vi "Begin.vi"(8 "error in":errorcluster) -> (0 "error out":errorcluster)   [LabVIEW 2015]
doc: "Called before other user functions, this VI is expected to open initial I/O refnums, load in file data, and do all program initialization. Notice that the <B>error out</B> terminal is simply used for data flow. Wiring it to other structures or subVIs ensures that this VI runs first."
uses:
  <vilib>/Rock Robotics/WPI/DriverStation/WPI_DriverStationRobotMode2.ctl
  <vilib>/Rock Robotics/SystemInterfaces/DIO/FPGA_DIOPWMChannel.ctl
  <vilib>/Rock Robotics/WPI/SafetyOutput/WPI_SafetyOutputConfigMenu.ctl
  <vilib>/Rock Robotics/WPI/Joystick/WPI_JoystickDeviceEnum.ctl
  <vilib>/Rock Robotics/WPI/Solenoid/WPI_SolenoidChannel.ctl
  <vilib>/Rock Robotics/SystemInterfaces/DIO/FPGA_DIOChannel.ctl
  <vilib>/Rock Robotics/SystemInterfaces/DIO/FPGA_DIORelayChannel.ctl
  <vilib>/Rock Robotics/SystemInterfaces/spilib/spi_bus.ctl
  Robot Global Data.vi
  <vilib>/Rock Robotics/WPI/RobotDrive/WPI_RobotDriveOpen2MotorWithVictor.vi
  <vilib>/Rock Robotics/WPI/MotorControl/WPI_MotorControlOpen Victor.vi
  <vilib>/Rock Robotics/WPI/MotorControl/WPI_MotorControlOpen SPARK.vi
  <vilib>/Rock Robotics/WPI/Counter/WPI_CounterDigitalInputToDigitalSource.vi
  <vilib>/Rock Robotics/WPI/Counter/WPI_CounterOpen UpDown Mode.vi
  <vilib>/Rock Robotics/WPI/Solenoid/WPI_SolenoidOpenDouble.vi
  <vilib>/Rock Robotics/WPI/Gyro/WPI_GyroXRS450_SPI_Open.vi
  Robot Global.vi
  <vilib>/Rock Robotics/WPI/Accelerometer/InternalAccelerometer/WPI_AccelerometerInternalOpen.vi
  <vilib>/Rock Robotics/SystemInterfaces/AI/FPGA_AIChannel.ctl
  <vilib>/Rock Robotics/Network Tables/NT Write String Array.vi
  <vilib>/Rock Robotics/SystemInterfaces/AI/FPGA_AIGyroChannel.ctl
  <vilib>/Rock Robotics/WPI/Solenoid/WPI_SolenoidOpenSingle.vi
  <vilib>/Rock Robotics/WPI/Ultrasonic/WPI_SonarMB1010AnalogOpen.vi
  <vilib>/Rock Robotics/WPI/Gyro/WPI_GyroAnalogOpen.vi
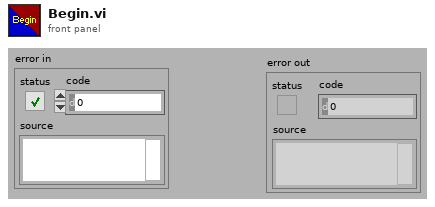
[diagram p1: front panel]
types:
  T1 = typedef "WPI_DriverStationRobotMode2.ctl" = enum16{"Autonomous Disabled", "Autonomous Enabled", "Teleop Disabled", "Teleop Enabled", "Disconnected", "Finish", "Test Disabled", "Test Enabled", "Emergency Stopped"}
  T2 = typedef "FPGA_DIOChannel.ctl" = enum8{"DIO 0", "DIO 1", "DIO 2", "DIO 3", "DIO 4", "DIO 5", "DIO 6", "DIO 7", "DIO 8", "DIO 9", "DIO MXP 0", "DIO MXP 1", "DIO MXP 2", "DIO MXP 3", "DIO MXP 4", "DIO MXP 5", "DIO MXP 6", "DIO MXP 7", "DIO MXP 8", "DIO MXP 9", "DIO MXP 10", "DIO MXP 11", "DIO MXP 12", "DIO MXP 13", "DIO MXP 14", "DIO MXP 15", "Invalid"}
  T3 = typedef "FPGA_DIOPWMChannel.ctl" = enum8{"PWM 0", "PWM 1", "PWM 2", "PWM 3", "PWM 4", "PWM 5", "PWM 6", "PWM 7", "PWM 8", "PWM 9", "PWM MXP 0", "PWM MXP 1", "PWM MXP 2", "PWM MXP 3", "PWM MXP 4", "PWM MXP 5", "PWM MXP 6", "PWM MXP 7", "PWM MXP 8", "PWM MXP 9", "Invalid"}
  T4 = typedef "FPGA_AIChannel.ctl" = enum8{"AI 0", "AI 1", "AI 2", "AI 3", "AI MXP 0", "AI MXP 1", "AI MXP 2", "AI MXP 3", "Invalid"}
  T5 = typedef "WPI_JoystickDeviceEnum.ctl" = enum16{"USB 0", "USB 1", "USB 2", "USB 3", "USB 4", "USB 5"}
  T6 = typedef "WPI_SolenoidChannel.ctl" = enum8{"Solenoid 0", "Solenoid 1", "Solenoid 2", "Solenoid 3", "Solenoid 4", "Solenoid 5", "Solenoid 6", "Solenoid 7", "Invalid"}
  T7 = typedef "FPGA_AIGyroChannel.ctl" = enum8{"AI 0", "AI 1", "Invalid"}
  T8 = typedef "WPI_SafetyOutputConfigMenu.ctl" = enum16{"Enable", "Disable"}
  T9 = typedef "spi_bus.ctl" = enum16{"SPI On-Board, CS0", "SPI On-Board, CS1", "SPI On-Board, CS2", "SPI On-Board, CS3", "SPI MXP", "Invalid"}
  T10 = typedef "FPGA_DIORelayChannel.ctl" = enum8{"Relay 0", "Relay 1", "Relay 2", "Relay 3", "Invalid"}
  T11 = typedef "WPI_SolenoidDevRef.ctl" = cluster{"DevStatus":errorcluster, "Pneumatics Control Module":u8, "Forward Solenoid Channel":T6, "Reverse Solenoid Channel":T6}
  T12 = typedef "WPI_DigitalInputDevRef.ctl" = cluster{"DevStatus":errorcluster, "DIO Channel":T2}
  T13 = typedef "WPI_CompressorDevRef.ctl" = cluster{"DevStatus":errorcluster, "Pneumatics Control Module":u8}
  T14 = typedef "FPGA_CounterEncoderSourceConvertionLVSourceType.ctl" = cluster{"DevStatus":errorcluster, "AnalogTriggerMode?":bool, "DigitalMode":cluster{"DIO Channel":T15}, "AnalogTriggerMode":cluster{"AnalogTriggerIndex":T16, "OutputType":T17}}
  T15 = typedef "FPGA_DIODigitalSourceChannel.ctl" = enum8{"DIO 0", "DIO 1", "DIO 2", "DIO 3", "DIO 4", "DIO 5", "DIO 6", "DIO 7", "DIO 8", "DIO 9", "DIO MXP 0", "DIO MXP 1", "DIO MXP 2", "DIO MXP 3", "DIO MXP 4", "DIO MXP 5", "DIO MXP 6", "DIO MXP 7", "DIO MXP 8", "DIO MXP 9", "DIO MXP 10", "DIO MXP 11", "DIO MXP 12", "DIO MXP 13", "DIO MXP 14", "DIO MXP 15", "Disabled"}
  T16 = typedef "FPGA_AnalogTriggerIndex.ctl" = enum8{"Trig 0", "Trig 1", "Trig 2", "Trig 3", "Trig 4", "Trig 5", "Trig 6", "Trig 7", "Invalid"}
  T17 = typedef "FPGA_AnalogTriggerOutType.ctl" = enum16{"InWindow", "TriggerState", "Rising", "Falling"}
  T18 = typedef "WPI_RobotDriveDevRef.ctl" = cluster{"DevStatus":errorcluster, "Motors[]":T19[], "Square Inputs":bool, "Max Output":dbl}
  T19 = typedef "WPI_MotorControlDeviceRef.ctl" = cluster{"DeviceStatus":errorcluster, "Type":T20, "PWM":cluster{"PWM Channel":T3, "DeadBand":T21}, "CAN":cluster{"Device Number":u8, "Control Mode":T22, "Semaphore":T23, "Max Vout":dbl, "TalonSRX Control Mode":T24}, "Invert":bool}
  T20 = typedef "WPI_MotorControlType.ctl" = enum16{"PWM", "CAN", "CANTalonSRX"}
  T21 = typedef "WPI_PWMDeadband.ctl" = cluster{"Name":string, "maxPositivePwm":i32, "minPositivePwm":i32, "centerPwm":i32, "maxNegativePwm":i32, "minNegativePwm":i32, "angularRange":u16}
  T22 = typedef "WPI_CANJaguar_ControlMode.ctl" = enum8{"Percent VBus", "Current", "Speed", "Position", "Voltage"}
  T23 = typedef "Semaphore RefNum" = refnum<k1>
  T24 = typedef "WPI_CANTalonSRX_APIControlMode.ctl" = enum8{"Percent VBus", "Speed", "Position", "Slave", "Unchanged / Invalid", "Voltage Compensation", "Current", "Motion Profile"}
  T25 = typedef "WPI_SonarMB1010AnalogDeviceRef.ctl" = cluster{"AIDeviceRef":T26, "Scaling factor (V/in)":dbl, "Average Bits":u8}
  T26 = typedef "WPI_AnalogChannelDevRef.ctl" = cluster{"DevStatus":errorcluster, "Analog Channel":T4}
  T27 = typedef "WPI_GyroDevRef.ctl" = cluster{"DevStatus":errorcluster, "Analog Channel":T4, "Offset":dbl, "Gain (VoltsPerDegree/Second)":dbl, "Gyro Type":enum16{"Analog", "XRS450"}, "Handle":i32, "SPI Bus":T9, "Device Found":bool, "Sample Rate":dbl, "Calibrate On Open":bool}
  T28 = typedef "WPI_JoystickDevRef.ctl" = cluster{"Device":T5}
  T29 = typedef "WPI_EncoderDevRef.ctl" = cluster{"DevStatus":errorcluster, "EncoderIndex":T30, "CounterIndex":T31, "DistancePerCount":dbl, "Decoding Type":T32}
  T30 = typedef "FPGA_EncoderIdx.ctl" = enum8{"Enc 0", "Enc 1", "Enc 2", "Enc 3", "Enc 4", "Enc 5", "Enc 6", "Enc 7", "Invalid"}
  T31 = typedef "FPGA_CounterCtrSystemIndex.ctl" = enum8{"Ctr 0", "Ctr 1", "Ctr 2", "Ctr 3", "Ctr 4", "Ctr 5", "Ctr 6", "Ctr 7", "Invalid"}
  T32 = typedef "WPI_EncoderType.ctl" = enum16{"1x", "2x", "4x"}
  T33 = typedef "Robot Drive.ctl" = cluster{"RobotDriveDevRef":T18, "Joysticks":cluster{"JoystickDevRef":T28, "JoystickDevRef 2":T28}, "Sensor":T34, "Pneumatics":T42, "Defenses":cluster{"LeftArm MotorControlDeviceRef":T19, "RightArm MotorControlDeviceRef":T19}, "Hanging":cluster{"Left Erection MotorControlDeviceRef":T19, "Right Erection MotorControlDeviceRef":T19}, "Aquisition + Scoring":T43, "DigitalOutputDevRef":T46, "DigitalInputDevRef":T12}
  T34 = typedef "Sensors.ctl" = cluster{"GyroDevRef":T27, "Left Arm Limit DigitalInputDevRef":T12, "Right Arm Limit DigitalInputDevRef":T12, "Left Arm EncoderDevRef":T29, "Right Arm EncoderDevRef":T29, "Left Drive EncoderDevRef":T29, "Right Drive EncoderDevRef":T29, "BoB Photoeye DigitalInputDevRef":T12, "Range SonarMB1010AnalogDevRef":T25, "Shooter CounterDevRef":T35, "AccelerometerDevRef":T36, "Left Hanging Erecter EncoderDevRef":T29, "Right Hanging Erecter EncoderDevRef":T29, "TestDigitalInputDevRef":T12}
  T35 = typedef "WPI_CounterDevRef.ctl" = cluster{"DevStatus":errorcluster, "CntIndex":T31}
  T36 = typedef "WPI_AccelerometerDevRef.ctl" = cluster{"DevStatus":errorcluster, "Scaling":T37, "Analog Channels":T38, "I2C Bus":T39, "SPI Bus":T9, "Accel Range":T40, "ADXL Axes":T41, "Handle":i32, "Device Address":u8, "Accel Type":enum16{"Analog", "ADXL345 I2C", "ADXL345 SPI", "Internal", "ADXL362 SPI"}}
  T37 = typedef "WPI_AccelerometerScaling.ctl" = cluster{"Gain (VoltsPerG)":dbl, "Center Voltage":dbl}
  T38 = typedef "WPI_AccelerometerAnalogChannels.ctl" = cluster{"X-Axis":T4, "Y-Axis":T4, "Z-Axis":T4}
  T39 = typedef "i2c_bus.ctl" = enum16{"I2C On-Board", "I2C MXP", "Invalid"}
  T40 = typedef "ADXL345 Range.ctl" = u8
  T41 = typedef "WPI_AccelerometerADXL345 Axes.ctl" = cluster{"X-Axis":bool, "Y-Axis":bool, "Z-Axis":bool}
  T42 = typedef "Pnematics.ctl" = cluster{"CompressorDevRef":T13, "High and Low Gear DoubleSolenoidDevRef":T11, "PTO SolenoidDevRef":T11, "Hang Pin SolenoidDevRef":T11}
  T43 = typedef "Acquisition & Scoring.ctl" = cluster{"Outer Roller MotorControlDeviceRef":T19, "Inner Roller MotorControlDeviceRef":T19, "Scoring Top MotorControlDeviceRef":T19, "Scoring Bottom MotorControlDeviceRef":T19, "Flashlight RelayDevRef":T44}
  T44 = typedef "WPI_RelayDevRef.ctl" = cluster{"DevStatus":errorcluster, "Relay Channel":T10, "Relay Direction":T45}
  T45 = typedef "WPI_RelayDirection.ctl" = enum16{"Both directions", "Forward only", "Reverse only"}
  T46 = typedef "WPI_DigitalOutputDevRef.ctl" = cluster{"DIO Channel":T2, "DevStatus":errorcluster}
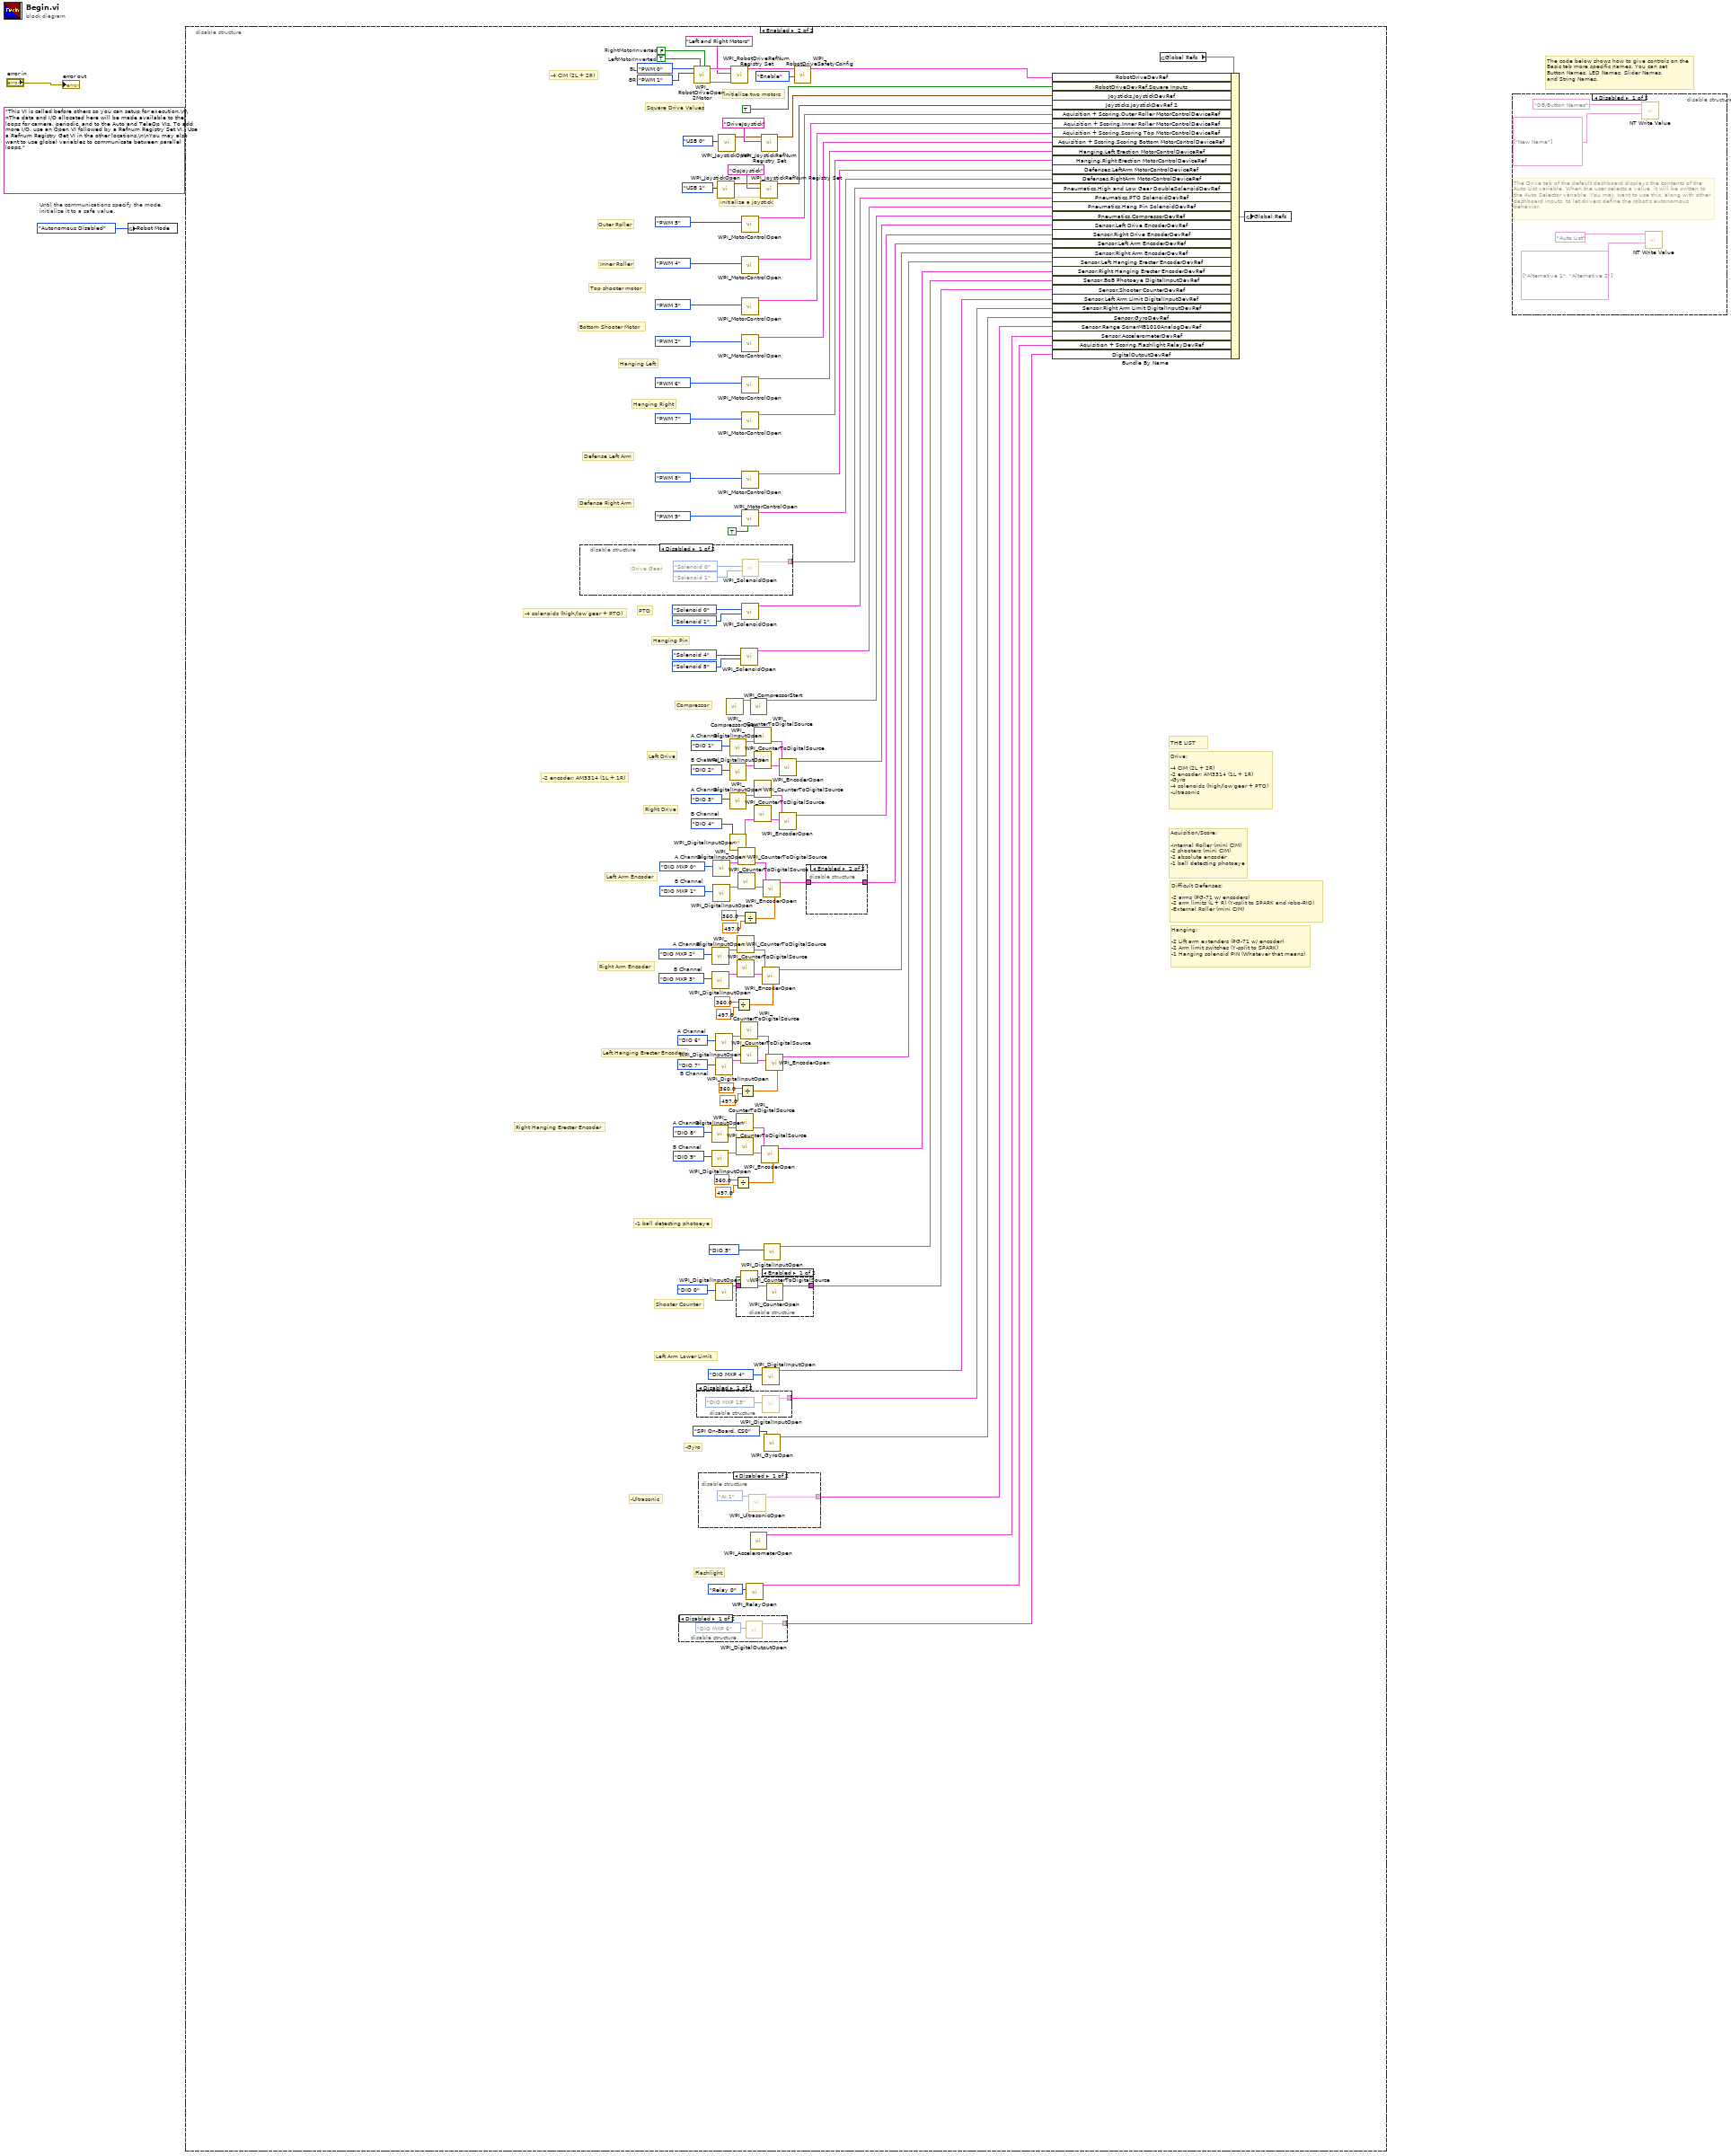
[diagram p0: block diagram]
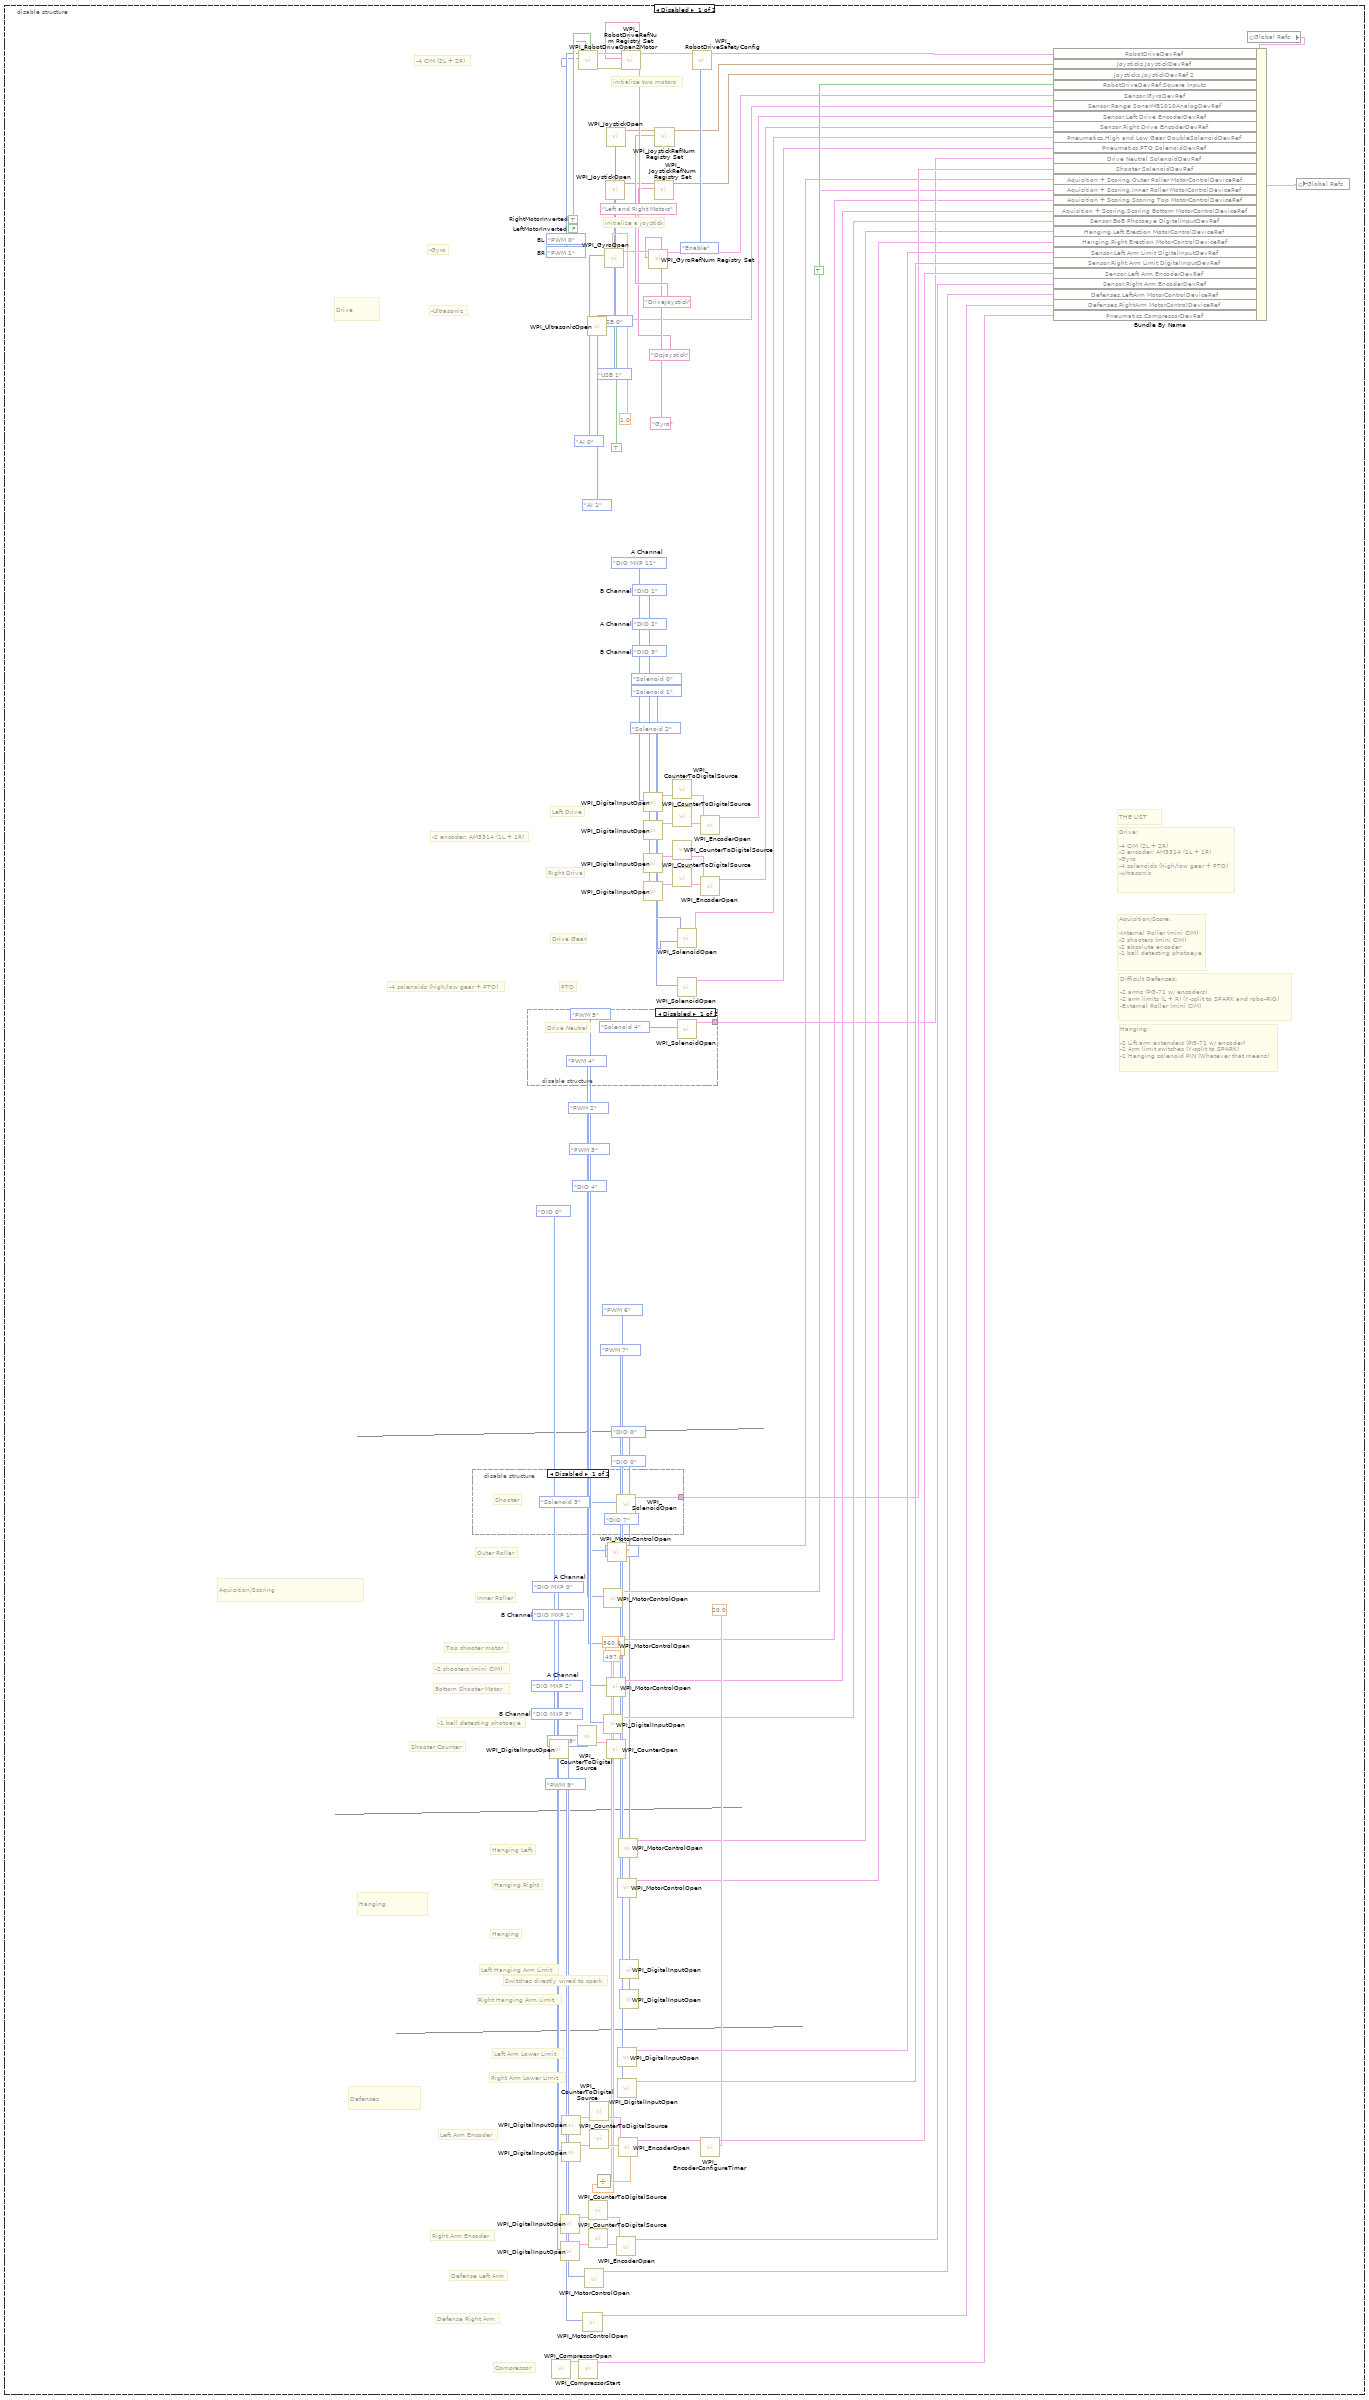
[diagram p2: hidden frame]
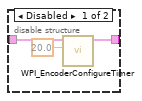
[diagram p10: hidden frame]
diagram:
  (unwired) "This VI is called before others so you can setup for execution.\n\nThe data and I/O allocated here will be made available to the loops for camera, periodic, and to the Auto and TeleOp VIs. To add more I/O, use an Open VI followed by a Refnum Registry Set VI.  Use a Refnum Registry Get VI in the other locations.\n\nYou may also want to use global variables to communicate between parallel loops."
  # "Until the communications specify the mode,\ninitialize it to a safe value."
  # "The code below shows how to give controls on the\nBasic tab more specific names. You can set\nButton Names, LED Names, Slider Names,\nand String Names."
  n1 = global write "Robot Global Data.vi" "Robot Mode"(WPI_DriverStationRobotMode2."Autonomous Disabled" ("Robot Mode")) -> ()
  n2 = disable-structure shown="Enabled" {
    frame Disabled {
      w39 = FPGA_DIOChannel."DIO 3"  # B Channel
      w38 = FPGA_DIOChannel."DIO 2"  # A Channel
      w45 = FPGA_DIOChannel."DIO 1"  # B Channel
      w44 = FPGA_DIOChannel."DIO MXP 11"  # A Channel
      w53 = FPGA_DIOChannel."DIO MXP 3"  # B Channel
      w52 = FPGA_DIOChannel."DIO MXP 2"  # A Channel
      w59 = FPGA_DIOChannel."DIO MXP 1"  # B Channel
      w58 = FPGA_DIOChannel."DIO MXP 0"  # A Channel
      w94 = FPGA_DIOPWMChannel."PWM 1"  # BR
      w95 = FPGA_DIOPWMChannel."PWM 0"  # BL
      w99 = FALSE  # LeftMotorInverted
      w100 = TRUE  # RightMotorInverted
      # "Switches directly wired to spark"
      # "Right Hanging Arm Limit"
      # "Left Hanging Arm Limit"
      # "Compressor"
      # "Shooter Counter"
      # "Inner Roller"
      # "Hanging"
      # "Defenses"
      # "Outer Roller"
      # "Hanging"
      # "Hanging Left"
      # "-1 ball detecting photoeye"
      # "-2 shooters (mini CIM)"
      # "Aquisition/Scoring"
      # "-4 solenoids (high/low gear + PTO)"
      # "-2 encoder: AM3314 (1L + 1R)"
      # "-Ultrasonic"
      # "-Gyro"
      # "-4 CIM (2L + 2R)"
      # "Hanging:\n\n-2 Lift arm extenders (PG-71 w/ encoder)\n-2 Arm limit switches (Y-split to SPARK)\n-1 Hanging solenoid PIN (Whatever that means)"
      # "Difficult Defenses:\n\n-2 arms (PG-71 w/ encoders)\n-2 arm limits (L + R) (Y-split to SPARK and robo-RIO)\n-External Roller (mini CIM)"
      # "Aquisition/Score:\n\n-Internal Roller (mini CIM)\n-2 shooters (mini CIM)\n-2 absolute encoder\n-1 ball detecting photoeye"
      # "Drive: \n\n-4 CIM (2L + 2R)\n-2 encoder: AM3314 (1L + 1R)\n-Gyro\n-4 solenoids (high/low gear + PTO)\n-ultrasonic"
      # "THE LIST"
      # "Drive"
      # "Right Drive"
      # "Left Drive"
      # "Right Arm Encoder"
      # "Left Arm Encoder"
      # "Right Arm Lower Limit"
      # "Left Arm Lower Limit"
      # "Hanging Right"
      # "Defense Right Arm"
      # "Defense Left Arm"
      # "PTO"
      # "Drive Gear"
      # "Top shooter motor"
      # "Bottom Shooter Motor"
      # "initialize a joystick"
      # "initialize two motors"
      n3 = disable-structure shown="Disabled" {
        disable-tunnel: [w103 _] -> w22
        frame Disabled {
          # "Shooter"
          n4 = call-poly <vilib>:"WPI_SolenoidOpen.vi"("Solenoid Channel"=WPI_SolenoidChannel."Solenoid 3") -> ("SolenoidDevRef"=w103:T11)  [unwired: 9 in, 1 out]
        }
        frame Enabled {
        }
      }
      n5 = disable-structure shown="Disabled" {
        disable-tunnel: [w101 _] -> w21
        frame Disabled {
          # "Drive Neutral"
          n6 = call-poly <vilib>:"WPI_SolenoidOpen.vi"("Solenoid Channel"=WPI_SolenoidChannel."Solenoid 4") -> ("SolenoidDevRef"=w101:T11)  [unwired: 9 in, 1 out]
        }
        frame Enabled {
        }
      }
      n7 = call <vilib>:"WPI_DigitalInputOpen.vi"("DIO Channel"=FPGA_DIOChannel."DIO 0" ("Source")) -> ("DigitalInputDevRef"=w6:T12)  [unwired: 1 in, 9 out]
      n8 = call <vilib>:"WPI_CompressorOpen.vi"() -> ("CompressorDevRef"=w76:T13)  [unwired: 14 in, 1 out]
      n9 = call <vilib>:"WPI_DigitalInputOpen.vi"("DIO Channel"=w52) -> ("DigitalInputDevRef"=w49:T12)  [unwired: 1 in, 9 out]
      n10 = call <vilib>:"WPI_DigitalInputOpen.vi"("DIO Channel"=w53) -> ("DigitalInputDevRef"=w50:T12)  [unwired: 1 in, 9 out]
      n11 = call <vilib>:"WPI_DigitalInputOpen.vi"("DIO Channel"=w58) -> ("DigitalInputDevRef"=w55:T12)  [unwired: 1 in, 9 out]
      n12 = call <vilib>:"WPI_DigitalInputOpen.vi"("DIO Channel"=w59) -> ("DigitalInputDevRef"=w56:T12)  [unwired: 1 in, 9 out]
      n13 = call-poly <vilib>:"WPI_CounterToDigitalSource.vi"("DigitalInputDevRef"=w6) -> ("Digital Source"=w8:T14)  [unwired: 6 out]
      n14 = call-poly <vilib>:"WPI_RobotDriveOpen2Motor.vi"("Right Motor Inverted"=w100, "Left Motor Inverted"=w99, "Right Motor"=w94, "Left Motor"=w95) -> ("error out"=w96:errorcluster, "RobotDriveDevRef"=w98:T18)  [unwired: 6 in]
      n15 = call <vilib>:"WPI_CompressorStart.vi"("CompressorDevRef"=w76) -> ("CompressorDevRef"=w5:T13)  [unwired: 9 in, 1 out]
      n16 = call-poly <vilib>:"WPI_MotorControlOpen.vi"("PWM Channel"=FPGA_DIOPWMChannel."PWM 9") -> ("MotorControlDeviceRef"=w25:T19)  [unwired: 9 in, 1 out]
      n17 = call-poly <vilib>:"WPI_MotorControlOpen.vi"("PWM Channel"=FPGA_DIOPWMChannel."PWM 8") -> ("MotorControlDeviceRef"=w26:T19)  [unwired: 9 in, 1 out]
      n18 = call-poly <vilib>:"WPI_UltrasonicOpen.vi"("Analog Channel"=FPGA_AIChannel."AI 1") -> ("SonarMB1010AnalogDevRef"=w16:T25)  [unwired: 9 in, 1 out]
      n19 = call-poly <vilib>:"WPI_CounterToDigitalSource.vi"("DigitalInputDevRef"=w49) -> ("Digital Source"=w48:T14)  [unwired: 6 out]
      n20 = call-poly <vilib>:"WPI_CounterToDigitalSource.vi"("DigitalInputDevRef"=w50) -> ("Digital Source"=w51:T14)  [unwired: 6 out]
      n21 = call-poly <vilib>:"WPI_CounterToDigitalSource.vi"("DigitalInputDevRef"=w55) -> ("Digital Source"=w54:T14)  [unwired: 6 out]
      n22 = call-poly <vilib>:"WPI_CounterToDigitalSource.vi"("DigitalInputDevRef"=w56) -> ("Digital Source"=w57:T14)  [unwired: 6 out]
      n23 = Divide(x=360.0, y=497.0) -> (x/y=w31:dbl)
      n24 = call-poly <vilib>:"WPI_MotorControlOpen.vi"("PWM Channel"=FPGA_DIOPWMChannel."PWM 4") -> ("MotorControlDeviceRef"=w9:T19)  [unwired: 9 in, 1 out]
      n25 = call <vilib>:"WPI_DigitalInputOpen.vi"("DIO Channel"=FPGA_DIOChannel."DIO 4") -> ("DigitalInputDevRef"=w24:T12)  [unwired: 9 in, 1 out]
      n26 = call-poly <vilib>:"WPI_GyroOpen.vi"("Calibration Time (s)"=1.0, "Calibrate On Open"=TRUE, "Analog Channel"=FPGA_AIGyroChannel."AI 0") -> ("GyroDevRef"=w82:T27)  [unwired: 6 in, 2 out]
      n27 = call-poly <vilib>:"WPI_MotorControlOpen.vi"("PWM Channel"=FPGA_DIOPWMChannel."PWM 2") -> ("MotorControlDeviceRef"=w15:T19)  [unwired: 9 in, 1 out]
      n28 = call <vilib>:"WPI_JoystickOpen.vi"("JoystickDevice"=WPI_JoystickDeviceEnum."USB 1") -> ("JoystickDevRef"=w63:T28)  [unwired: 10 in]
      n29 = call <vilib>:"WPI_JoystickOpen.vi"("JoystickDevice"=WPI_JoystickDeviceEnum."USB 0") -> ("JoystickDevRef"=w90:T28)  [unwired: 10 in]
      n30 = call-poly <vilib>:"WPI_MotorControlOpen.vi"("PWM Channel"=FPGA_DIOPWMChannel."PWM 3") -> ("MotorControlDeviceRef"=w23:T19)  [unwired: 9 in, 1 out]
      n31 = call-poly <vilib>:"WPI_CounterOpen.vi"("Up Source"=w8) -> ()  [unwired: 6 in, 5 out]
      n32 = call-poly <vilib>:"WPI_MotorControlOpen.vi"("PWM Channel"=FPGA_DIOPWMChannel."PWM 5") -> ("MotorControlDeviceRef"=w10:T19)  [unwired: 9 in, 1 out]
      n33 = call <vilib>:"WPI_EncoderOpen.vi"("BSource"=w51, "ASource"=w48) -> ("EncoderDevRef"=w46:T29)  [unwired: 6 in, 3 out]
      n34 = call-poly <vilib>:"WPI_MotorControlOpen.vi"("PWM Channel"=FPGA_DIOPWMChannel."PWM 7") -> ("MotorControlDeviceRef"=w12:T19)  [unwired: 9 in, 1 out]
      n35 = call <vilib>:"WPI_DigitalInputOpen.vi"("DIO Channel"=FPGA_DIOChannel."DIO 7") -> ("DigitalInputDevRef"=w66:T12)  [unwired: 9 in, 1 out]
      n36 = call <vilib>:"WPI_DigitalInputOpen.vi"("DIO Channel"=FPGA_DIOChannel."DIO 8") -> ("DigitalInputDevRef"=w65:T12)  [unwired: 9 in, 1 out]
      n37 = call-poly <vilib>:"WPI_MotorControlOpen.vi"("PWM Channel"=FPGA_DIOPWMChannel."PWM 6") -> ("MotorControlDeviceRef"=w13:T19)  [unwired: 9 in, 1 out]
      n38 = call <vilib>:"WPI_EncoderOpen.vi"("DistancePerCount"=w31, "BSource"=w57, "ASource"=w54) -> ("EncoderDevRef"=w47:T29)  [unwired: 5 in, 3 out]
      n39 = call <vilib>:"WPI_DigitalInputOpen.vi"("DIO Channel"=FPGA_DIOChannel."DIO 0") -> ()  [unwired: 9 in, 2 out]
      n40 = call <vilib>:"WPI_DigitalInputOpen.vi"("DIO Channel"=FPGA_DIOChannel."DIO 0") -> ()  [unwired: 9 in, 2 out]
      n41 = call <vilib>:"WPI_RobotDriveRefNum Registry Set.vi"("error in (no error)"=w96, "refnum name"="Left and Right Motors", "RobotDriveDevRef"=w98) -> ("RobotDriveDevRef"=w93:T18)  [unwired: 1 in, 7 out]
      n42 = call <vilib>:"WPI_DigitalInputOpen.vi"("DIO Channel"=w44) -> ("DigitalInputDevRef"=w41:T12)  [unwired: 1 in, 9 out]
      n43 = call <vilib>:"WPI_DigitalInputOpen.vi"("DIO Channel"=w45) -> ("DigitalInputDevRef"=w42:T12)  [unwired: 1 in, 9 out]
      n44 = call <vilib>:"WPI_DigitalInputOpen.vi"("DIO Channel"=w38) -> ("DigitalInputDevRef"=w35:T12)  [unwired: 1 in, 9 out]
      n45 = call <vilib>:"WPI_DigitalInputOpen.vi"("DIO Channel"=w39) -> ("DigitalInputDevRef"=w36:T12)  [unwired: 1 in, 9 out]
      n46 = call <vilib>:"WPI_GyroRefNum Registry Set.vi"("refnum name"="Gyro", "GyroDevRef"=w82) -> ("GyroDevRef"=w80:T27)  [unwired: 8 in, 1 out]
      n47 = call <vilib>:"WPI_JoystickRefNum Registry Set.vi"("refnum name"="OpJoystick", "JoystickDevRef"=w63) -> ("JoystickDevRef"=w60:T28)  [unwired: 8 in, 1 out]
      n48 = call <vilib>:"WPI_JoystickRefNum Registry Set.vi"("refnum name"="DriveJoystick", "JoystickDevRef"=w90) -> ("JoystickDevRef"=w61:T28)  [unwired: 8 in, 1 out]
      n49 = call-poly <vilib>:"WPI_CounterToDigitalSource.vi"("DigitalInputDevRef"=w41) -> ("Digital Source"=w40:T14)  [unwired: 6 out]
      n50 = call-poly <vilib>:"WPI_CounterToDigitalSource.vi"("DigitalInputDevRef"=w42) -> ("Digital Source"=w43:T14)  [unwired: 6 out]
      n51 = call-poly <vilib>:"WPI_CounterToDigitalSource.vi"("DigitalInputDevRef"=w35) -> ("Digital Source"=w34:T14)  [unwired: 6 out]
      n52 = call-poly <vilib>:"WPI_CounterToDigitalSource.vi"("DigitalInputDevRef"=w36) -> ("Digital Source"=w37:T14)  [unwired: 6 out]
      n53 = call-poly <vilib>:"WPI_SolenoidOpen.vi"("Solenoid Channel"=WPI_SolenoidChannel."Solenoid 2") -> ("SolenoidDevRef"=w20:T11)  [unwired: 9 in, 1 out]
      n54 = call-poly <vilib>:"WPI_SolenoidOpen.vi"("Reverse Solenoid Channel"=WPI_SolenoidChannel."Solenoid 1", "Forward Solenoid Channel"=WPI_SolenoidChannel."Solenoid 0") -> ("SolenoidDevRef"=w19:T11)  [unwired: 8 in, 1 out]
      n55 = call <vilib>:"WPI_RobotDriveSafetyConfig.vi"("mode"=WPI_SafetyOutputConfigMenu."Enable", "RobotDriveDevRef"=w93) -> ("RobotDriveDevRef"=w87:T18)  [unwired: 8 in, 1 out]
      n56 = call <vilib>:"WPI_EncoderOpen.vi"("BSource"=w43, "ASource"=w40) -> ("EncoderDevRef"=w17:T29)  [unwired: 6 in, 3 out]
      n57 = call <vilib>:"WPI_EncoderOpen.vi"("BSource"=w37, "ASource"=w34) -> ("EncoderDevRef"=w18:T29)  [unwired: 6 in, 3 out]
      n58 = call <vilib>:"WPI_EncoderConfigureTimer.vi"("Minimum Rate"=20.0, "EncoderDevRef"=w47) -> ("EncoderDevRef"=w33:T29)  [unwired: 8 in, 1 out]
      n59 = global read "Robot Global.vi" "Global Refs"() -> (w88:T33)
      n60 = Bundle By Name(cluster=w88, "RobotDriveDevRef"=w87, "Joysticks.JoystickDevRef"=w61, "Joysticks.JoystickDevRef 2"=w60, "RobotDriveDevRef.Square Inputs"=TRUE, "Sensor.GyroDevRef"=w80, "Sensor.Range SonarMB1010AnalogDevRef"=w16, "Sensor.Left Drive EncoderDevRef"=w17, "Sensor.Right Drive EncoderDevRef"=w18, "Pneumatics.High and Low Gear DoubleSolenoidDevRef"=w19, "Pneumatics.PTO SolenoidDevRef"=w20, "Drive Neutral SolenoidDevRef"=w21, "Shooter SolenoidDevRef"=w22, "Aquisition + Scoring.Outer Roller MotorControlDeviceRef"=w10, "Aquisition + Scoring.Inner Roller MotorControlDeviceRef"=w9, "Aquisition + Scoring.Scoring Top MotorControlDeviceRef"=w15, "Aquisition + Scoring.Scoring Bottom MotorControlDeviceRef"=w23, "Sensor.BoB Photoeye DigitalInputDevRef"=w24, "Hanging.Left Erection MotorControlDeviceRef"=w13, "Hanging.Right Erection MotorControlDeviceRef"=w12, "Sensor.Left Arm Limit DigitalInputDevRef"=w66, "Sensor.Right Arm Limit DigitalInputDevRef"=w65, "Sensor.Left Arm EncoderDevRef"=w33, "Sensor.Right Arm EncoderDevRef"=w46, "Defenses.LeftArm MotorControlDeviceRef"=w26, "Defenses.RightArm MotorControlDeviceRef"=w25, "Pneumatics.CompressorDevRef"=w5) -> (w86:T33)
      n61 = global write "Robot Global.vi" "Global Refs"(w86) -> ()
    }
    frame Enabled {
      w121 = FPGA_DIOChannel."DIO MXP 3"  # B Channel
      w120 = FPGA_DIOChannel."DIO MXP 2"  # A Channel
      w125 = FPGA_DIOChannel."DIO MXP 1"  # B Channel
      w124 = FPGA_DIOChannel."DIO MXP 0"  # A Channel
      w137 = FPGA_DIOChannel."DIO 9"  # B Channel
      w136 = FPGA_DIOChannel."DIO 8"  # A Channel
      w146 = FPGA_DIOChannel."DIO 7"  # B Channel
      w145 = FPGA_DIOChannel."DIO 6"  # A Channel
      w159 = FPGA_DIOChannel."DIO 4"  # B Channel
      w158 = FPGA_DIOChannel."DIO 3"  # A Channel
      w165 = FPGA_DIOChannel."DIO 2"  # B Channel
      w164 = FPGA_DIOChannel."DIO 1"  # A Channel
      w215 = FPGA_DIOPWMChannel."PWM 1"  # BR
      w216 = FPGA_DIOPWMChannel."PWM 0"  # BL
      w220 = TRUE  # LeftMotorInverted
      w221 = FALSE  # RightMotorInverted
      # "Right Arm Encoder"
      # "Left Arm Encoder"
      # "-4 solenoids (high/low gear + PTO)"
      # "Flashlight"
      # "Right Hanging Erecter Encoder"
      # "Left Hanging Erecter Encoder"
      # "Hanging Pin"
      # "Compressor"
      # "Shooter Counter"
      # "Inner Roller"
      # "Outer Roller"
      # "Hanging Left"
      # "-1 ball detecting photoeye"
      # "-2 encoder: AM3314 (1L + 1R)"
      # "-Ultrasonic"
      # "-Gyro"
      # "Right Drive"
      # "Left Drive"
      # "Left Arm Lower Limit"
      # "Hanging Right"
      # "Defense Right Arm"
      # "Defense Left Arm"
      # "PTO"
      # "Top shooter motor"
      # "Bottom Shooter Motor"
      # "Square Drive Values"
      # "-4 CIM (2L + 2R)"
      # "Hanging:\n\n-2 Lift arm extenders (PG-71 w/ encoder)\n-2 Arm limit switches (Y-split to SPARK)\n-1 Hanging solenoid PIN (Whatever that means)"
      # "Difficult Defenses:\n\n-2 arms (PG-71 w/ encoders)\n-2 arm limits (L + R) (Y-split to SPARK and robo-RIO)\n-External Roller (mini CIM)"
      # "Aquisition/Score:\n\n-Internal Roller (mini CIM)\n-2 shooters (mini CIM)\n-2 absolute encoder\n-1 ball detecting photoeye"
      # "Drive: \n\n-4 CIM (2L + 2R)\n-2 encoder: AM3314 (1L + 1R)\n-Gyro\n-4 solenoids (high/low gear + PTO)\n-ultrasonic"
      # "THE LIST"
      # "initialize a joystick"
      # "initialize two motors"
      n62 = disable-structure shown="Disabled" {
        disable-tunnel: [w226 _] -> w194
        frame Disabled {
          # "Drive Gear"
          n63 = call-poly <vilib>:"WPI_SolenoidOpen.vi"("Reverse Solenoid Channel"=WPI_SolenoidChannel."Solenoid 1", "Forward Solenoid Channel"=WPI_SolenoidChannel."Solenoid 0") -> ("SolenoidDevRef"=w226:T11)  [unwired: 8 in, 1 out]
        }
        frame Enabled {
        }
      }
      n64 = disable-structure shown="Disabled" {
        disable-tunnel: [w229 _] -> w176
        frame Disabled {
          n65 = call <vilib>:"WPI_DigitalOutputOpen.vi"("DIO Channel"=FPGA_DIOChannel."DIO MXP 6") -> ("DigitalOutputDevRef"=w229:T46)  [unwired: 9 in, 1 out]
        }
        frame Enabled {
        }
      }
      n66 = call-poly <vilib>:"WPI_RobotDriveOpen2Motor.vi"("Right Motor Inverted"=w221, "Left Motor Inverted"=w220, "Right Motor"=w215, "Left Motor"=w216) -> ("error out"=w217:errorcluster, "RobotDriveDevRef"=w219:T18)  [unwired: 6 in]
      n67 = disable-structure shown="Disabled" {
        disable-tunnel: [w231 _] -> w184
        frame Disabled {
          n68 = call <vilib>:"WPI_DigitalInputOpen.vi"("DIO Channel"=FPGA_DIOChannel."DIO MXP 15") -> ("DigitalInputDevRef"=w231:T12)  [unwired: 9 in, 1 out]
        }
        frame Enabled {
        }
      }
      n69 = disable-structure shown="Disabled" {
        disable-tunnel: [w233 _] -> w183
        frame Disabled {
          n70 = call-poly <vilib>:"WPI_UltrasonicOpen.vi"("Analog Channel"=FPGA_AIChannel."AI 1") -> ("SonarMB1010AnalogDevRef"=w233:T25)  [unwired: 9 in, 1 out]
        }
        frame Enabled {
        }
      }
      n71 = call <vilib>:"WPI_DigitalInputOpen.vi"("DIO Channel"=w136) -> ("DigitalInputDevRef"=w133:T12)  [unwired: 1 in, 9 out]
      n72 = call <vilib>:"WPI_DigitalInputOpen.vi"("DIO Channel"=w137) -> ("DigitalInputDevRef"=w134:T12)  [unwired: 1 in, 9 out]
      n73 = call <vilib>:"WPI_DigitalInputOpen.vi"("DIO Channel"=w120) -> ("DigitalInputDevRef"=w111:T12)  [unwired: 1 in, 9 out]
      n74 = call <vilib>:"WPI_DigitalInputOpen.vi"("DIO Channel"=w121) -> ("DigitalInputDevRef"=w110:T12)  [unwired: 1 in, 9 out]
      n75 = call <vilib>:"WPI_DigitalInputOpen.vi"("DIO Channel"=w124) -> ("DigitalInputDevRef"=w108:T12)  [unwired: 1 in, 9 out]
      n76 = call <vilib>:"WPI_DigitalInputOpen.vi"("DIO Channel"=w125) -> ("DigitalInputDevRef"=w109:T12)  [unwired: 1 in, 9 out]
      n77 = call <vilib>:"WPI_DigitalInputOpen.vi"("DIO Channel"=w145) -> ("DigitalInputDevRef"=w142:T12)  [unwired: 1 in, 9 out]
      n78 = call <vilib>:"WPI_DigitalInputOpen.vi"("DIO Channel"=w146) -> ("DigitalInputDevRef"=w143:T12)  [unwired: 1 in, 9 out]
      n79 = call <vilib>:"WPI_DigitalInputOpen.vi"("DIO Channel"=FPGA_DIOChannel."DIO 0" ("Source")) -> ("DigitalInputDevRef"=w149:T12)  [unwired: 1 in, 9 out]
      n80 = call <vilib>:"WPI_JoystickOpen.vi"("JoystickDevice"=WPI_JoystickDeviceEnum."USB 1") -> ("JoystickDevRef"=w208:T28)  [unwired: 10 in]
      n81 = call <vilib>:"WPI_JoystickOpen.vi"("JoystickDevice"=WPI_JoystickDeviceEnum."USB 0") -> ("JoystickDevRef"=w211:T28)  [unwired: 10 in]
      n82 = call <vilib>:"WPI_CompressorOpen.vi"() -> ("CompressorDevRef"=w172:T13)  [unwired: 14 in, 1 out]
      n83 = call <vilib>:"WPI_DigitalInputOpen.vi"("DIO Channel"=w164) -> ("DigitalInputDevRef"=w161:T12)  [unwired: 1 in, 9 out]
      n84 = call <vilib>:"WPI_DigitalInputOpen.vi"("DIO Channel"=w165) -> ("DigitalInputDevRef"=w162:T12)  [unwired: 1 in, 9 out]
      n85 = call <vilib>:"WPI_DigitalInputOpen.vi"("DIO Channel"=w158) -> ("DigitalInputDevRef"=w155:T12)  [unwired: 1 in, 9 out]
      n86 = call <vilib>:"WPI_DigitalInputOpen.vi"("DIO Channel"=w159) -> ("DigitalInputDevRef"=w156:T12)  [unwired: 1 in, 9 out]
      n87 = call <vilib>:"WPI_RobotDriveRefNum Registry Set.vi"("error in (no error)"=w217, "refnum name"="Left and Right Motors", "RobotDriveDevRef"=w219) -> ("RobotDriveDevRef"=w214:T18)  [unwired: 1 in, 7 out]
      n88 = Divide(x=360.0, y=497.0) -> (x/y=w129:dbl)
      n89 = Divide(x=360.0, y=497.0) -> (x/y=w112:dbl)
      n90 = call-poly <vilib>:"WPI_CounterToDigitalSource.vi"("DigitalInputDevRef"=w133) -> ("Digital Source"=w132:T14)  [unwired: 6 out]
      n91 = call-poly <vilib>:"WPI_CounterToDigitalSource.vi"("DigitalInputDevRef"=w134) -> ("Digital Source"=w135:T14)  [unwired: 6 out]
      n92 = disable-structure shown="Enabled" {
        disable-tunnel: [w224 w225] -> w105
        disable-tunnel: w149 -> [w222 w225]
        frame Enabled {
          n93 = call-poly <vilib>:"WPI_CounterToDigitalSource.vi"("DigitalInputDevRef"=w222) -> ("Digital Source"=w223:T14)  [unwired: 6 out]
          n94 = call-poly <vilib>:"WPI_CounterOpen.vi"("Up Source"=w223) -> ("CounterDevRef"=w224:T35)  [unwired: 6 in, 4 out]
        }
        frame Disabled {
        }
      }
      n95 = call-poly <vilib>:"WPI_CounterToDigitalSource.vi"("DigitalInputDevRef"=w111) -> ("Digital Source"=w118:T14)  [unwired: 6 out]
      n96 = call-poly <vilib>:"WPI_CounterToDigitalSource.vi"("DigitalInputDevRef"=w110) -> ("Digital Source"=w119:T14)  [unwired: 6 out]
      n97 = call-poly <vilib>:"WPI_CounterToDigitalSource.vi"("DigitalInputDevRef"=w108) -> ("Digital Source"=w122:T14)  [unwired: 6 out]
      n98 = call-poly <vilib>:"WPI_CounterToDigitalSource.vi"("DigitalInputDevRef"=w109) -> ("Digital Source"=w123:T14)  [unwired: 6 out]
      n99 = Divide(x=360.0, y=497.0) -> (x/y=w138:dbl)
      n100 = call-poly <vilib>:"WPI_SolenoidOpen.vi"("Reverse Solenoid Channel"=WPI_SolenoidChannel."Solenoid 5", "Forward Solenoid Channel"=WPI_SolenoidChannel."Solenoid 4" ("Solenoid Channel")) -> ("SolenoidDevRef"=w192:T11)  [unwired: 8 in, 1 out]
      n101 = call-poly <vilib>:"WPI_CounterToDigitalSource.vi"("DigitalInputDevRef"=w142) -> ("Digital Source"=w141:T14)  [unwired: 6 out]
      n102 = call-poly <vilib>:"WPI_CounterToDigitalSource.vi"("DigitalInputDevRef"=w143) -> ("Digital Source"=w144:T14)  [unwired: 6 out]
      n103 = call-poly <vilib>:"WPI_MotorControlOpen.vi"("PWM Channel"=FPGA_DIOPWMChannel."PWM 5") -> ("MotorControlDeviceRef"=w202:T19)  [unwired: 9 in, 1 out]
      n104 = call-poly <vilib>:"WPI_MotorControlOpen.vi"("PWM Channel"=FPGA_DIOPWMChannel."PWM 4") -> ("MotorControlDeviceRef"=w201:T19)  [unwired: 9 in, 1 out]
      n105 = call-poly <vilib>:"WPI_MotorControlOpen.vi"("PWM Channel"=FPGA_DIOPWMChannel."PWM 3") -> ("MotorControlDeviceRef"=w200:T19)  [unwired: 9 in, 1 out]
      n106 = call-poly <vilib>:"WPI_MotorControlOpen.vi"("PWM Channel"=FPGA_DIOPWMChannel."PWM 2") -> ("MotorControlDeviceRef"=w199:T19)  [unwired: 9 in, 1 out]
      n107 = call-poly <vilib>:"WPI_MotorControlOpen.vi"("PWM Channel"=FPGA_DIOPWMChannel."PWM 6") -> ("MotorControlDeviceRef"=w198:T19)  [unwired: 9 in, 1 out]
      n108 = call-poly <vilib>:"WPI_MotorControlOpen.vi"("PWM Channel"=FPGA_DIOPWMChannel."PWM 7") -> ("MotorControlDeviceRef"=w197:T19)  [unwired: 9 in, 1 out]
      n109 = call-poly <vilib>:"WPI_MotorControlOpen.vi"("PWM Channel"=FPGA_DIOPWMChannel."PWM 8") -> ("MotorControlDeviceRef"=w196:T19)  [unwired: 9 in, 1 out]
      n110 = call-poly <vilib>:"WPI_MotorControlOpen.vi"("Invert"=TRUE, "PWM Channel"=FPGA_DIOPWMChannel."PWM 9") -> ("MotorControlDeviceRef"=w195:T19)  [unwired: 8 in, 1 out]
      n111 = call-poly <vilib>:"WPI_SolenoidOpen.vi"("Reverse Solenoid Channel"=WPI_SolenoidChannel."Solenoid 1", "Forward Solenoid Channel"=WPI_SolenoidChannel."Solenoid 0" ("Solenoid Channel")) -> ("SolenoidDevRef"=w193:T11)  [unwired: 8 in, 1 out]
      n112 = Divide(x=360.0, y=497.0) -> (x/y=w117:dbl)
      n113 = call <vilib>:"WPI_RelayOpen.vi"("Relay Channel"=FPGA_DIORelayChannel."Relay 0") -> ("RelayDevRef"=w177:T44)  [unwired: 9 in, 1 out]
      n114 = call <vilib>:"WPI_CompressorStart.vi"("CompressorDevRef"=w172) -> ("CompressorDevRef"=w191:T13)  [unwired: 9 in, 1 out]
      n115 = call-poly <vilib>:"WPI_AccelerometerOpen.vi"() -> ("AccelerometerDevRef"=w180:T36)  [unwired: 10 in, 1 out]
      n116 = call-poly <vilib>:"WPI_CounterToDigitalSource.vi"("DigitalInputDevRef"=w161) -> ("Digital Source"=w160:T14)  [unwired: 6 out]
      n117 = call-poly <vilib>:"WPI_CounterToDigitalSource.vi"("DigitalInputDevRef"=w162) -> ("Digital Source"=w163:T14)  [unwired: 6 out]
      n118 = call-poly <vilib>:"WPI_CounterToDigitalSource.vi"("DigitalInputDevRef"=w155) -> ("Digital Source"=w154:T14)  [unwired: 6 out]
      n119 = call-poly <vilib>:"WPI_CounterToDigitalSource.vi"("DigitalInputDevRef"=w156) -> ("Digital Source"=w157:T14)  [unwired: 6 out]
      n120 = call <vilib>:"WPI_JoystickRefNum Registry Set.vi"("refnum name"="OpJoystick", "JoystickDevRef"=w208) -> ("JoystickDevRef"=w203:T28)  [unwired: 8 in, 1 out]
      n121 = call <vilib>:"WPI_JoystickRefNum Registry Set.vi"("refnum name"="DriveJoystick", "JoystickDevRef"=w211) -> ("JoystickDevRef"=w204:T28)  [unwired: 8 in, 1 out]
      n122 = call <vilib>:"WPI_EncoderOpen.vi"("DistancePerCount"=w129, "BSource"=w135, "ASource"=w132) -> ("EncoderDevRef"=w178:T29)  [unwired: 5 in, 3 out]
      n123 = call <vilib>:"WPI_EncoderOpen.vi"("DistancePerCount"=w112, "BSource"=w119, "ASource"=w118) -> ("EncoderDevRef"=w187:T29)  [unwired: 5 in, 3 out]
      n124 = call <vilib>:"WPI_DigitalInputOpen.vi"("DIO Channel"=FPGA_DIOChannel."DIO MXP 4") -> ("DigitalInputDevRef"=w185:T12)  [unwired: 9 in, 1 out]
      n125 = call <vilib>:"WPI_EncoderOpen.vi"("DistancePerCount"=w117, "BSource"=w123, "ASource"=w122) -> ("EncoderDevRef"=w175:T29)  [unwired: 5 in, 3 out]
      n126 = call <vilib>:"WPI_DigitalInputOpen.vi"("DIO Channel"=FPGA_DIOChannel."DIO 5") -> ("DigitalInputDevRef"=w186:T12)  [unwired: 9 in, 1 out]
      n127 = call-poly <vilib>:"WPI_GyroOpen.vi"("SPI Bus"=spi_bus."SPI On-Board, CS0") -> ("GyroDevRef"=w107:T27)  [unwired: 9 in, 1 out]
      n128 = call <vilib>:"WPI_EncoderOpen.vi"("DistancePerCount"=w138, "BSource"=w144, "ASource"=w141) -> ("EncoderDevRef"=w179:T29)  [unwired: 5 in, 3 out]
      n129 = call <vilib>:"WPI_EncoderOpen.vi"("BSource"=w163, "ASource"=w160) -> ("EncoderDevRef"=w190:T29)  [unwired: 6 in, 3 out]
      n130 = call <vilib>:"WPI_EncoderOpen.vi"("BSource"=w157, "ASource"=w154) -> ("EncoderDevRef"=w189:T29)  [unwired: 6 in, 3 out]
      n131 = call <vilib>:"WPI_RobotDriveSafetyConfig.vi"("mode"=WPI_SafetyOutputConfigMenu."Enable", "RobotDriveDevRef"=w214) -> ("RobotDriveDevRef"=w182:T18)  [unwired: 8 in, 1 out]
      n132 = disable-structure shown="Enabled" {
        disable-tunnel: w175 -> [w237 w238]
        disable-tunnel: [w235 w238] -> w188
        frame Disabled {
          n133 = call <vilib>:"WPI_EncoderConfigureTimer.vi"("Minimum Rate"=20.0, "EncoderDevRef"=w237) -> ("EncoderDevRef"=w235:T29)  [unwired: 8 in, 1 out]
        }
        frame Enabled {
        }
      }
      n134 = global read "Robot Global.vi" "Global Refs"() -> (w206:T33)
      n135 = Bundle By Name(cluster=w206, "RobotDriveDevRef"=w182, "RobotDriveDevRef.Square Inputs"=TRUE, "Joysticks.JoystickDevRef"=w204, "Joysticks.JoystickDevRef 2"=w203, "Aquisition + Scoring.Outer Roller MotorControlDeviceRef"=w202, "Aquisition + Scoring.Inner Roller MotorControlDeviceRef"=w201, "Aquisition + Scoring.Scoring Top MotorControlDeviceRef"=w200, "Aquisition + Scoring.Scoring Bottom MotorControlDeviceRef"=w199, "Hanging.Left Erection MotorControlDeviceRef"=w198, "Hanging.Right Erection MotorControlDeviceRef"=w197, "Defenses.LeftArm MotorControlDeviceRef"=w196, "Defenses.RightArm MotorControlDeviceRef"=w195, "Pneumatics.High and Low Gear DoubleSolenoidDevRef"=w194, "Pneumatics.PTO SolenoidDevRef"=w193, "Pneumatics.Hang Pin SolenoidDevRef"=w192, "Pneumatics.CompressorDevRef"=w191, "Sensor.Left Drive EncoderDevRef"=w190, "Sensor.Right Drive EncoderDevRef"=w189, "Sensor.Left Arm EncoderDevRef"=w188, "Sensor.Right Arm EncoderDevRef"=w187, "Sensor.Left Hanging Erecter EncoderDevRef"=w179, "Sensor.Right Hanging Erecter EncoderDevRef"=w178, "Sensor.BoB Photoeye DigitalInputDevRef"=w186, "Sensor.Shooter CounterDevRef"=w105, "Sensor.Left Arm Limit DigitalInputDevRef"=w185, "Sensor.Right Arm Limit DigitalInputDevRef"=w184, "Sensor.GyroDevRef"=w107, "Sensor.Range SonarMB1010AnalogDevRef"=w183, "Sensor.AccelerometerDevRef"=w180, "Aquisition + Scoring.Flashlight RelayDevRef"=w177, "DigitalOutputDevRef"=w176) -> (w205:T33)
      n136 = global write "Robot Global.vi" "Global Refs"(w205) -> ()
    }
  }
  n137 = disable-structure shown="Disabled" {
    frame Disabled {
      # "The Drive tab of the default dashboard displays the contents of the\nAuto List variable. When the user selects a value, it will be written to\nthe Auto Selector variable. You may want to use this, along with other\ndashboard inputs, to let drivers define the robot's autonomous\nbehavior."
      n138 = call-poly <vilib>:"NT Write Value.vi"("String Array"=string[] ["New Name"], "Name"="DB/Button Names") -> ()  [unwired: 9 in, 1 out]
      n139 = call-poly <vilib>:"NT Write Value.vi"("String Array"=string[] ["Alternative 1", "Alternative 2"], "Name"="Auto List") -> ()  [unwired: 9 in, 1 out]
    }
    frame Enabled {
    }
  }
  "error out" <- "error in"
